vi "Adjust Gain and Phase.vi"(8 "error in (no error)":errorcluster, 11 "Sinusoidal Fit in":refnum<class "Sinusoidal Fit.lvclass">) -> (0 "error out":errorcluster, 3 "Sinusoidal Fit out":refnum<class "Sinusoidal Fit.lvclass">)   [LabVIEW 2016, in "Sinusoidal Fit.lvclass"]
uses:
  Sinusoidal Fit.lvclass
  Sinusoidal Fit.lvclass/Sinusoidal Fit.ctl
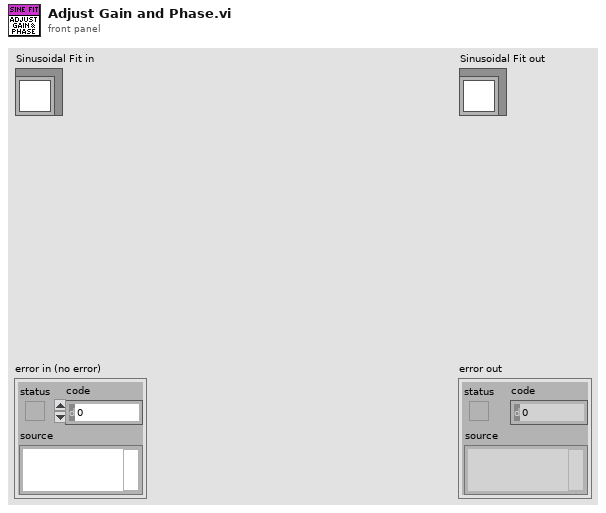
[diagram p1: front panel]
types:
  T1 = typedef "Typedef - Sinusoidal Fit Coefficients.ctl" = cluster{"Offset":dbl, "Gain":dbl, "Phase":dbl, "Freq":dbl}
  T2 = typedef "Typedef - Gain and Phase.ctl" = cluster{"Gain":dbl, "Gain SD":dbl, "Phase":dbl, "Phase SD":dbl}
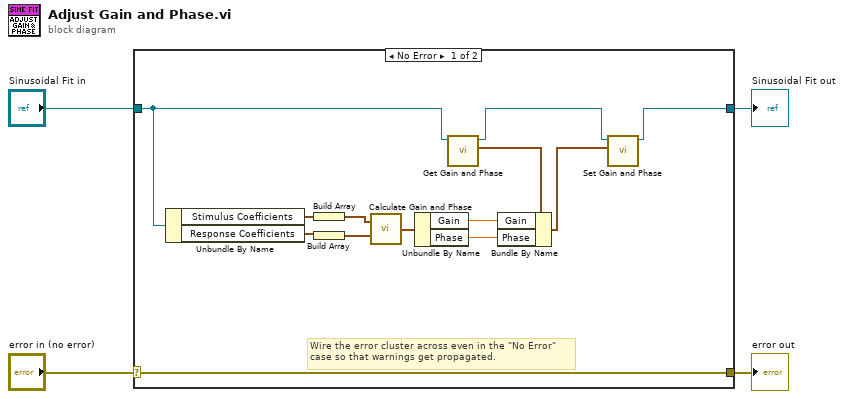
[diagram p0: block diagram]
diagram:
  n1 = case shown="No Error" "error in (no error)" {
    selector: "error in (no error)" -> [w17 w19]
    tunnel: [w17 w19] -> w3
    tunnel: [w5 w18] -> w1
    tunnel: "Sinusoidal Fit in" -> [w12 w18]
    frame No Error {
      # "Wire the error cluster across even in the \"No Error\"\ncase so that warnings get propagated."
      n2 = Unbundle By Name(w12) -> ("Stimulus Coefficients"=w16:T1, "Response Coefficients"=w14:T1)
      n3 = Build Array(w16) -> (w15:T1[])
      n4 = Build Array(w14) -> (w13:T1[])
      n5 = call "Calculate Gain and Phase.vi"("Response"=w13, "Stimulus"=w15) -> ("Gain and Phase out"=w10:T2)
      n6 = Unbundle By Name(w10) -> ("Gain"=w9:dbl, "Phase"=w8:dbl)
      n7 = call-dynamic "Get Gain and Phase.vi"("Sinusoidal Fit in"=w12) -> ("Gain and Phase"=w11:T2, "Sinusoidal Fit out"=w6:refnum<class "Sinusoidal Fit.lvclass">)  [unwired: 8 in, 1 out]
      n8 = Bundle By Name(cluster=w11, "Gain"=w9, "Phase"=w8) -> (w7:T2)
      n9 = call-dynamic "Set Gain and Phase.vi"("Gain and Phase"=w7, "Sinusoidal Fit in"=w6) -> ("Sinusoidal Fit out"=w5:refnum<class "Sinusoidal Fit.lvclass">)  [unwired: 8 in, 1 out]
    }
    frame Error {
    }
  }
  "error out" <- w3
  "Sinusoidal Fit out" <- w1
